vi "Write Console Options Ref.vi"(4 "Start Ref":refnum<vi>, 6 "Console Options":refnum<vi>[](array[refnum]), 11 "Entry Console View Definition in":refnum<class "Entry Console View Definition.lvclass">) -> (3 "Entry Console View Definition out":refnum<class "Entry Console View Definition.lvclass">)   [LabVIEW 2019, in "Entry Console View Definition.lvclass"]
uses:
  <vilib>/gpm_packages/@cs/Car-wash/Source/Entry Console View Definition/Entry Console View Definition/Entry Console View Definition.lvclass
  <vilib>/gpm_packages/@cs/Car-wash/Source/Entry Console View Definition/Entry Console View Definition/Entry Console View Definition.lvclass/Entry Console View Definition.ctl
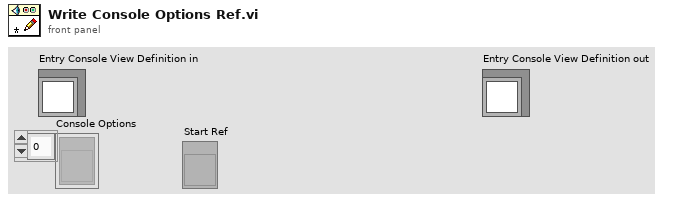
[diagram p1: front panel]
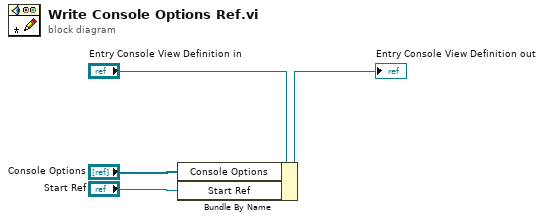
[diagram p0: block diagram]
diagram:
  n1 = Bundle By Name(cluster="Entry Console View Definition in", "Console Options"="Console Options", "Start Ref"="Start Ref") -> (→"Entry Console View Definition out":refnum<class "Entry Console View Definition.lvclass">)
